vi "Position Q Key.vi"(8 "error in (no error)":errorcluster, 10 "Zero Key":refnum<vi>, 11 "Q Key":refnum<vi>) -> (0 "error out":errorcluster)   [LabVIEW 2014]
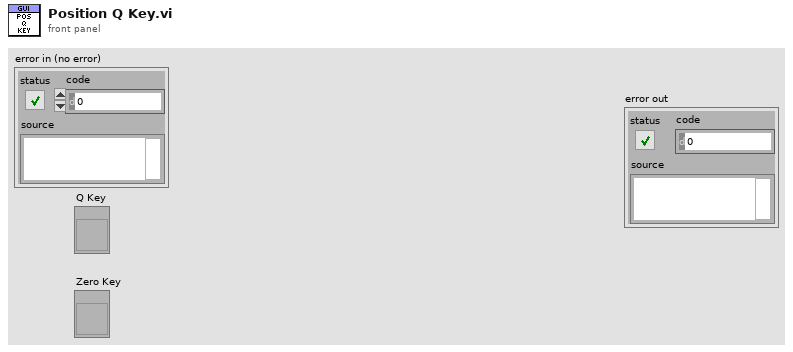
[diagram p1: front panel]
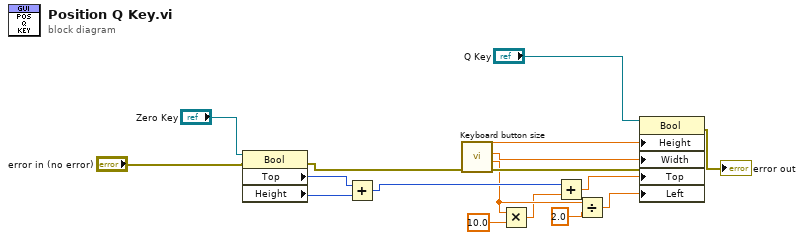
[diagram p0: block diagram]
diagram:
  n1 = property class="Bool"(reference="Zero Key", error in="error in (no error)") -> (error out=w9:errorcluster, "Top"=w7:i32, "Height"=w6:u32)  [unwired: 1 out]
  n2 = Add(x=w7, y=w6) -> (x+y=w5:u32)
  n3 = call "Keyboard button size.vi"("error in (no error)"=w9) -> ("error out"=w16:errorcluster, "Key Spacing"=w3:dbl, "Key Width"=w14:dbl, "Key Height"=w13:dbl)  [unwired: 7 in]
  n4 = Multiply(x=w3, y=10.0) -> (x*y=w1:dbl)
  n5 = Add(x=w5, y=w1) -> (x+y=w4:dbl)
  n6 = Divide(x=w3, y=2.0) -> (x/y=w11:dbl)
  n7 = property class="Bool"(reference="Q Key", error in=w16, "Height"=w13, "Width"=w14, "Top"=w4, "Left"=w11) -> (error out=→"error out":errorcluster)  [unwired: 1 out]
